vi "AnguloLimite.vi"(6 "XdoAttacker":dbl, 8 "atacando contra":bool, 9 "AnguloGol":dbl, 10 "IA State":T1={"our_robots"=[], "enemy_robots"=[], "balls"=[], "geometry"={"line_width"=0, "field_length"=0, "field_width"=0, "boundary_width"=0, "referee_width"=0, "goal_width"=0, "goal_depth"=0, "goal_wall_width"=0, "center_circle_radius"=0, "defense_radius"=0, "defense_stretch"=0, "free_kick_from_defense_dist"=0, "penalty_spot_from_field_line_dist"=0, "penalty_line_from_spot_dist"=0}, "IA Judge"={"stage"="", "command"="", "our_goalie_id"=0.0, "enemy_goalie_id"=0.0, "command enum"=enum."Halt", "Time"=enum."Azul"}, "Received Timestamp"=timestamp(0 s since 1904-01-01), "Events"={"Touch"=FALSE, "Ball out"=FALSE, "id touch"=0.0, "Ball out of \nVision"=FALSE, "Ball inside \nGoalie area"=FALSE, "Robot not responding"=FALSE, "Robots responding status"=[1.0, 1.0, 1.0, 1.0, 1.0, 1.0], "Enemy Ball \nPossession"=FALSE, "Pass State"=FALSE, "id end of pass"=0.0, "Kick"=FALSE, "Id ini Possession"=0.0, "Ball Possesion"=FALSE, "Id Possesion"=0.0}}, 11 "YdoAttacker":dbl) -> (1 "Angulo Limite":dbl)   [LabVIEW 2016]
uses:
  Core/AI Input.ctl
  Core/AI Robot.ctl
  Intel/Functions Enum.ctl
  Intel/AttackerStates.ctl
  Core/AI Ball.ctl
  Core/Field Size.ctl
  Core/AI Judge.ctl
  Intel/Command Enum.ctl
  Events/Events.ctl
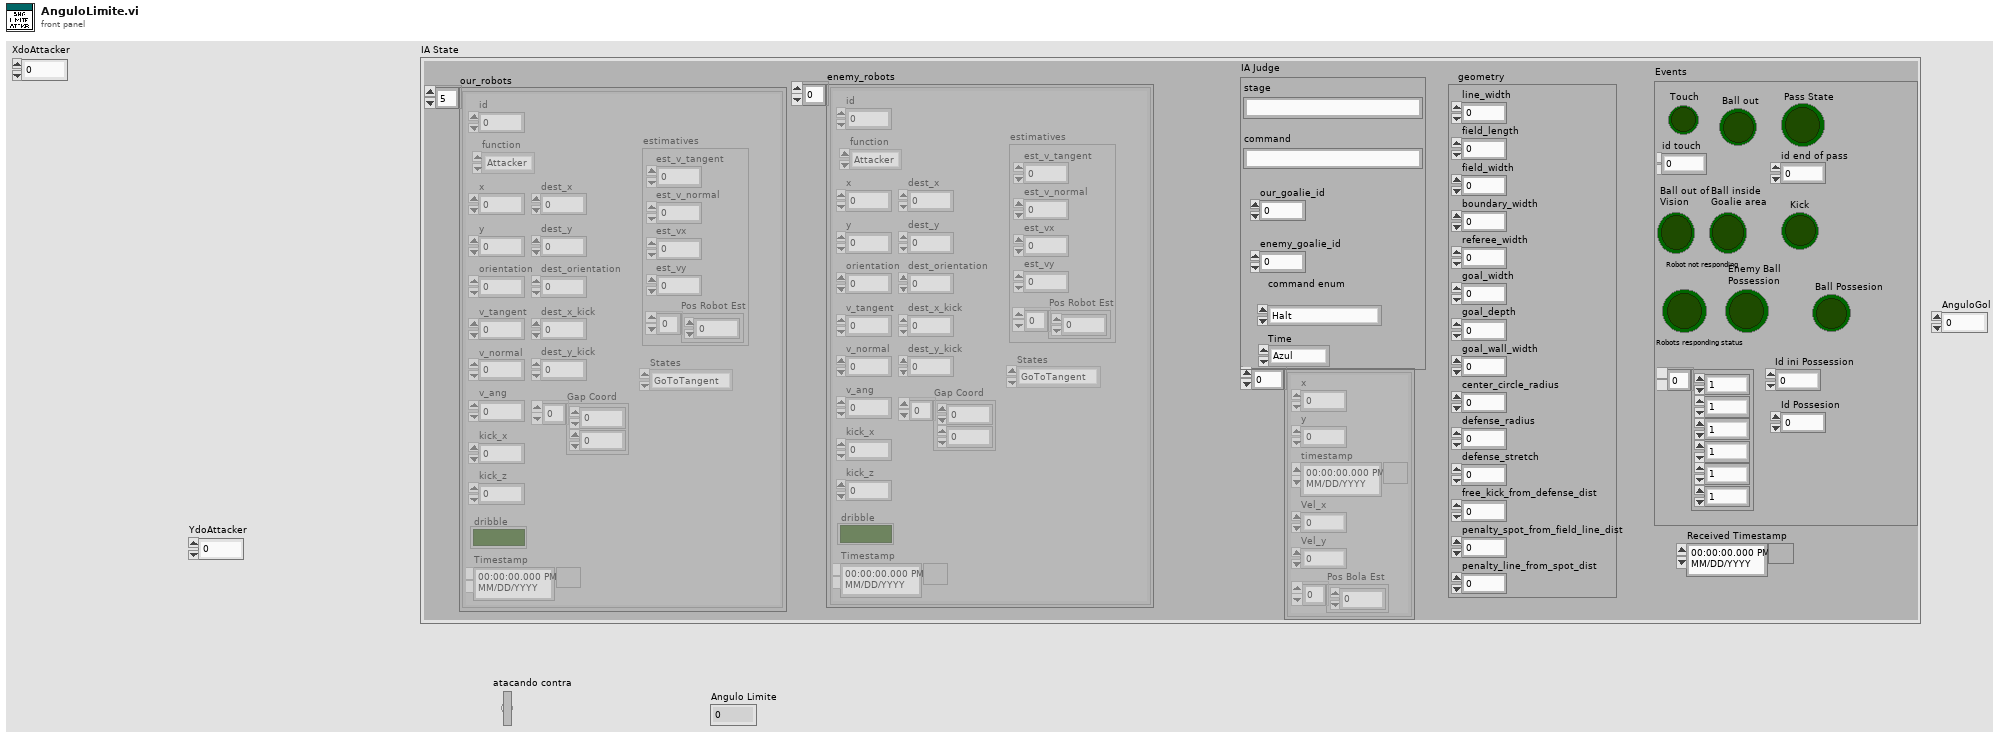
[diagram p1: front panel]
types:
  T1 = typedef "AI Input.ctl" = cluster{"our_robots":T2[], "enemy_robots":T2[], "balls":T5[], "geometry":T6, "IA Judge":T7, "Received Timestamp":timestamp, "Events":T9}
  T2 = typedef "AI Robot.ctl" = cluster{"id":u32, "function":T3, "x":dbl, "y":dbl, "orientation":dbl, "v_tangent":dbl, "v_normal":dbl, "v_ang":dbl, "kick_x":dbl, "kick_z":dbl, "dribble":bool, "Timestamp":timestamp, "dest_x":dbl, "dest_y":dbl, "dest_orientation":dbl, "estimatives":cluster{"est_v_tangent":dbl, "est_v_normal":dbl, "est_vx":dbl, "est_vy":dbl, "Pos Robot Est":dbl[]}, "dest_x_kick":dbl, "dest_y_kick":dbl, "Gap Coord":dbl[], "States":T4}
  T3 = typedef "Functions Enum.ctl" = enum16{"Attacker", "Goalie", "Defender", "Striker", "Goto 0", "Dummy", "Kicker", "ZigZag"}
  T4 = typedef "AttackerStates.ctl" = enum16{"Pass", "GoToTangent", "BallGetting", "GoToKick", ""}
  T5 = typedef "AI Ball.ctl" = cluster{"x":dbl, "y":dbl, "timestamp":timestamp, "Vel_x":dbl, "Vel_y":dbl, "Pos Bola Est":dbl[]}
  T6 = typedef "Field Size.ctl" = cluster{"line_width":u32, "field_length":u32, "field_width":u32, "boundary_width":u32, "referee_width":u32, "goal_width":u32, "goal_depth":u32, "goal_wall_width":u32, "center_circle_radius":u32, "defense_radius":u32, "defense_stretch":u32, "free_kick_from_defense_dist":u32, "penalty_spot_from_field_line_dist":u32, "penalty_line_from_spot_dist":u32}
  T7 = typedef "AI Judge.ctl" = cluster{"stage":string, "command":string, "our_goalie_id":dbl, "enemy_goalie_id":dbl, "command enum":T8, "Time":enum16{"Azul", "Amarelo"}}
  T8 = typedef "Command Enum.ctl" = enum16{"Halt", "Stop", "Force Start", "PKA Normal Start", "Prepare Kickoff Ally", "PKE Normal Start", "Prepare Kickoff Enemy", "Prepare Penalty Ally", "PPA Normal Start", "Prepare Penalty Enemy", "PPE Normal Start", "Direct Free Enemy", "Direct Free Ally", "Indirect Free Enemy", "Indirect Free Ally", "Timeout Enemy", "Timeout Ally", "Goal Enemy", "Goal Ally", "Ball Placement Enemy", "Ball Placement Ally", "Normal Half Time", "Extra Time Break", "Extra Half Time", "None", "Post Game"}
  T9 = typedef "Events.ctl" = cluster{"Touch":bool, "Ball out":bool, "id touch":dbl, "Ball out of \nVision":bool, "Ball inside \nGoalie area":bool, "Robot not responding":bool, "Robots responding status":dbl[], "Enemy Ball \nPossession":bool, "Pass State":bool, "id end of pass":dbl, "Kick":bool, "Id ini Possession":dbl, "Ball Possesion":bool, "Id Possesion":dbl}
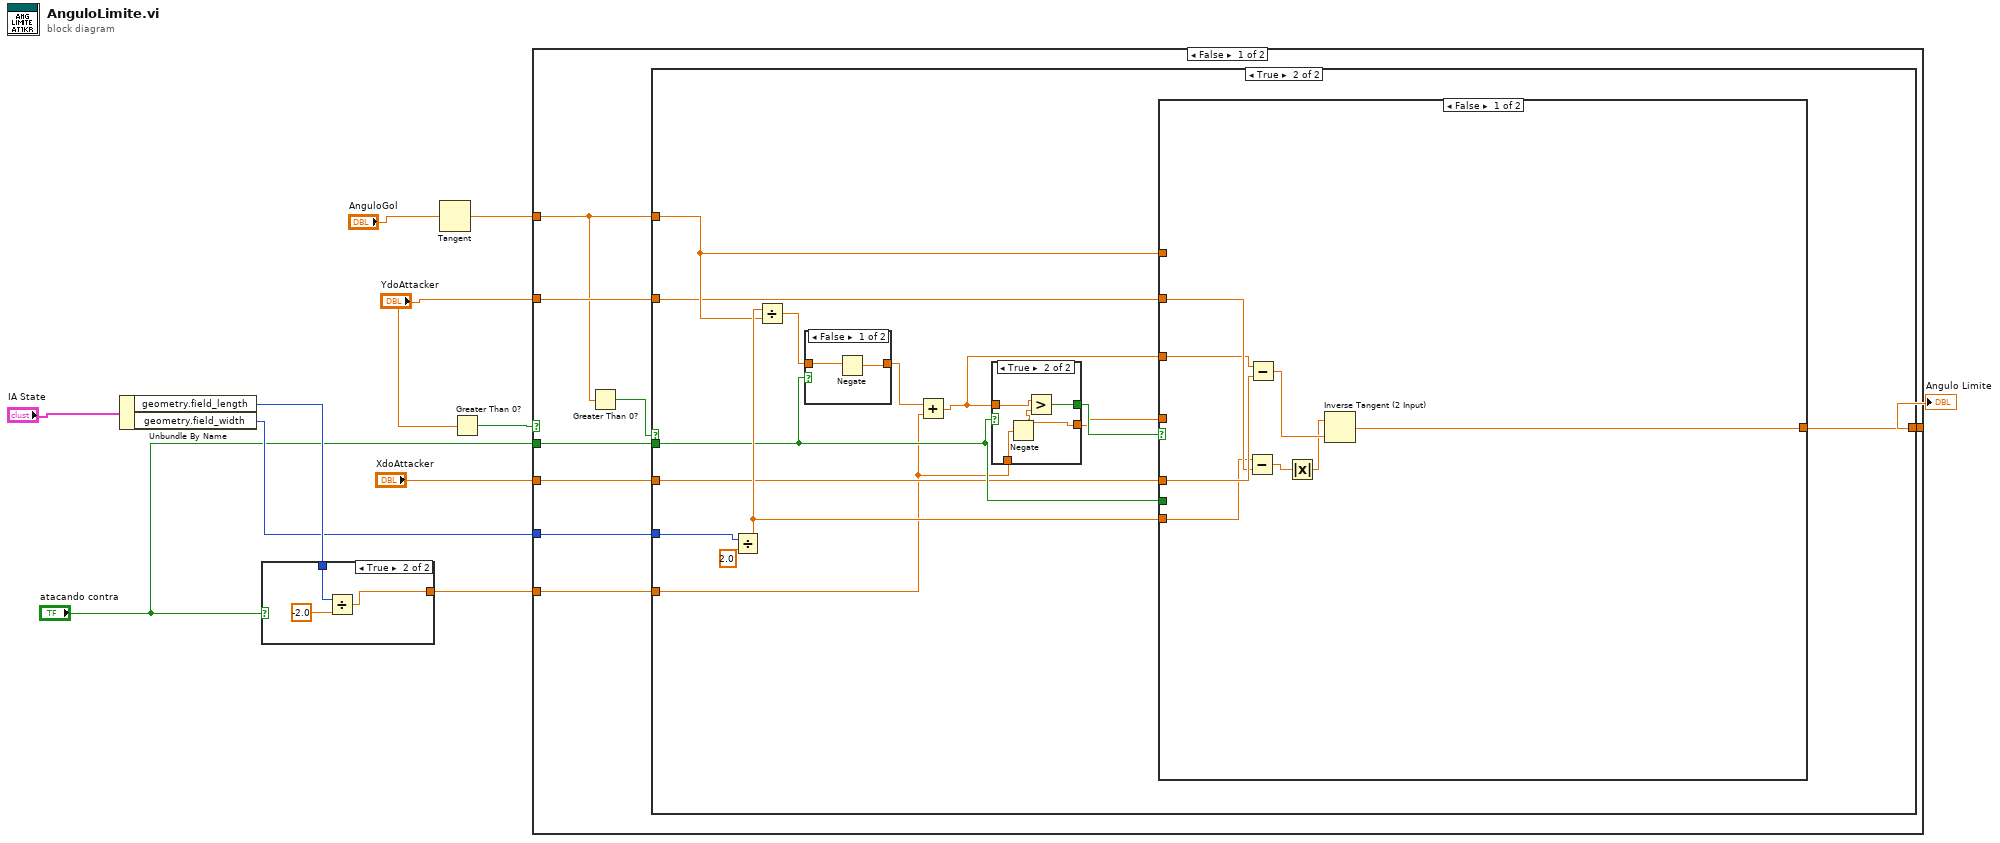
[diagram p0: block diagram]
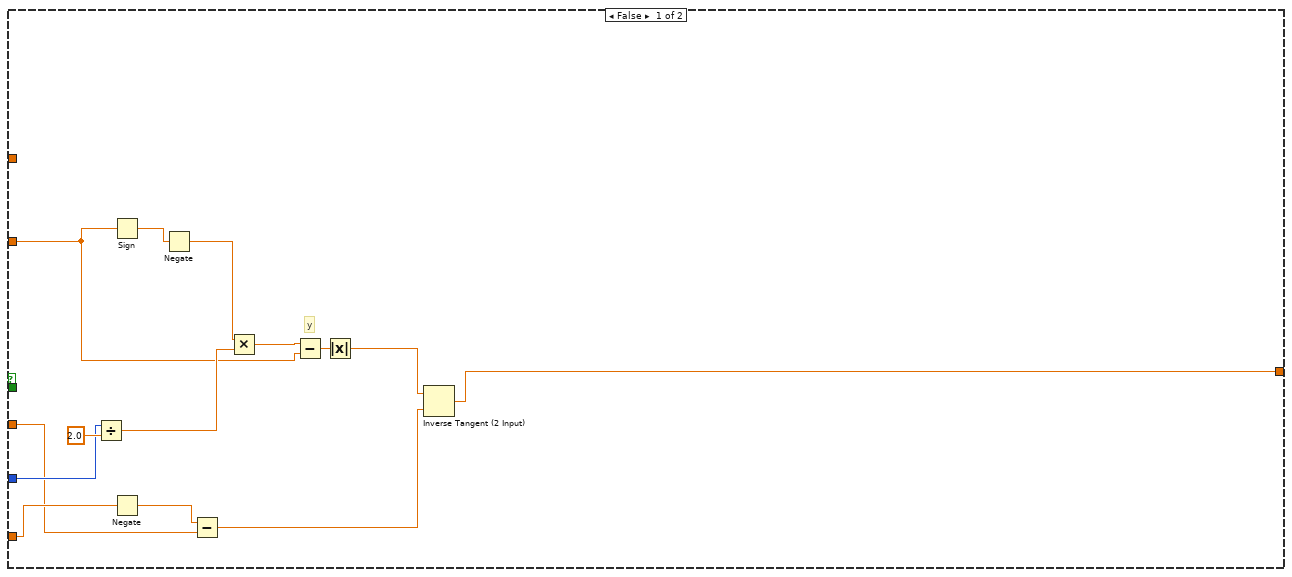
[diagram p2: hidden frame]
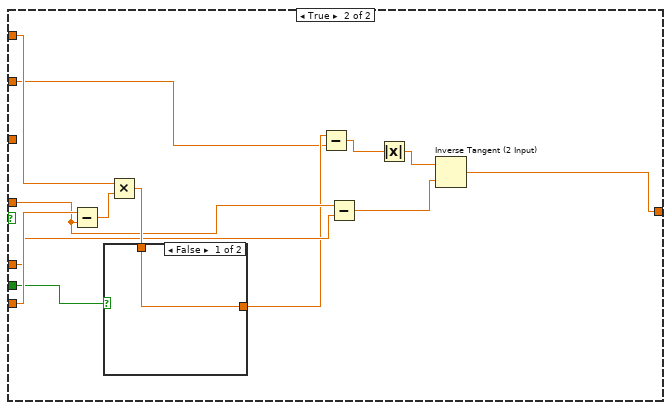
[diagram p3: hidden frame]
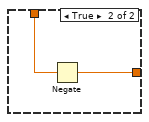
[diagram p4: hidden frame]
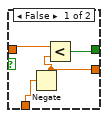
[diagram p5: hidden frame]
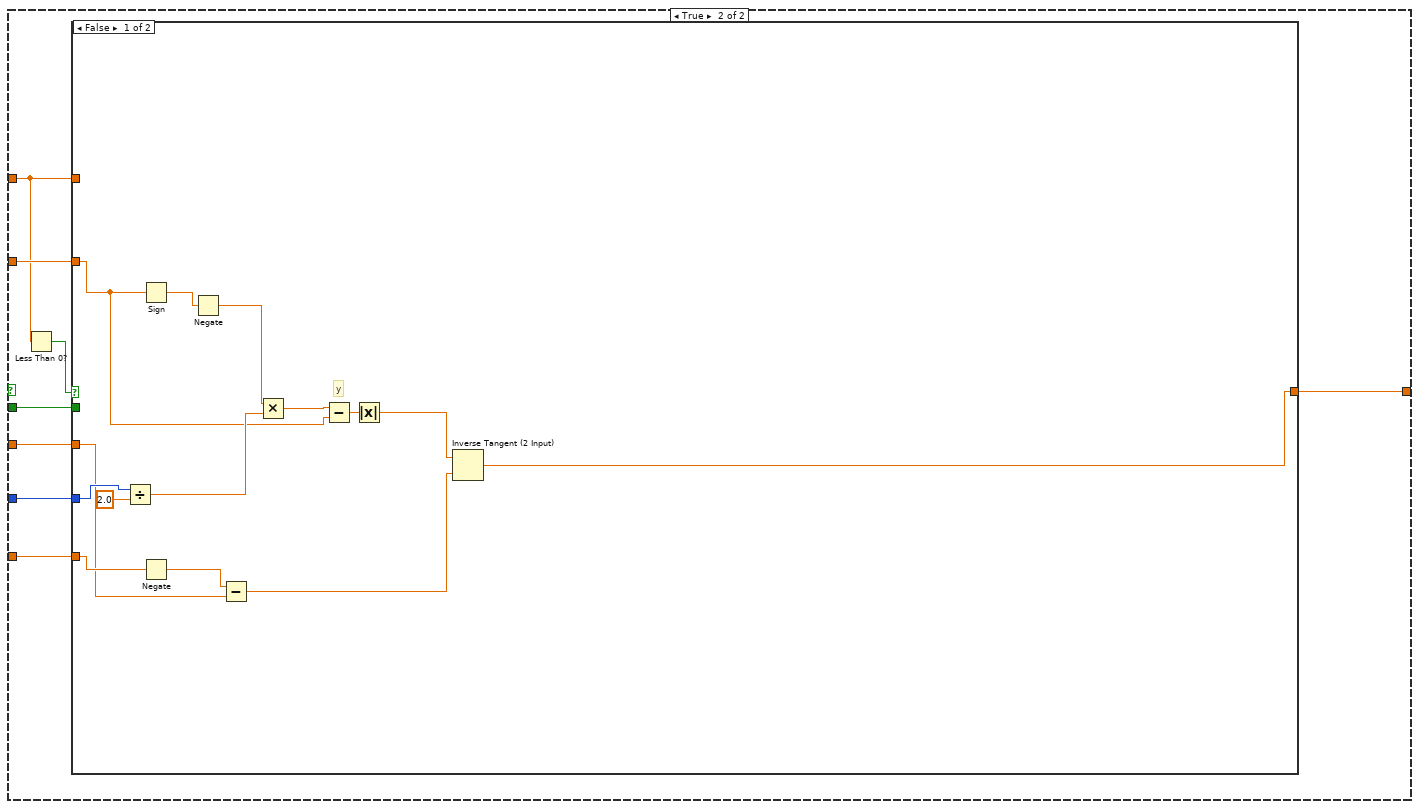
[diagram p7: hidden frame]
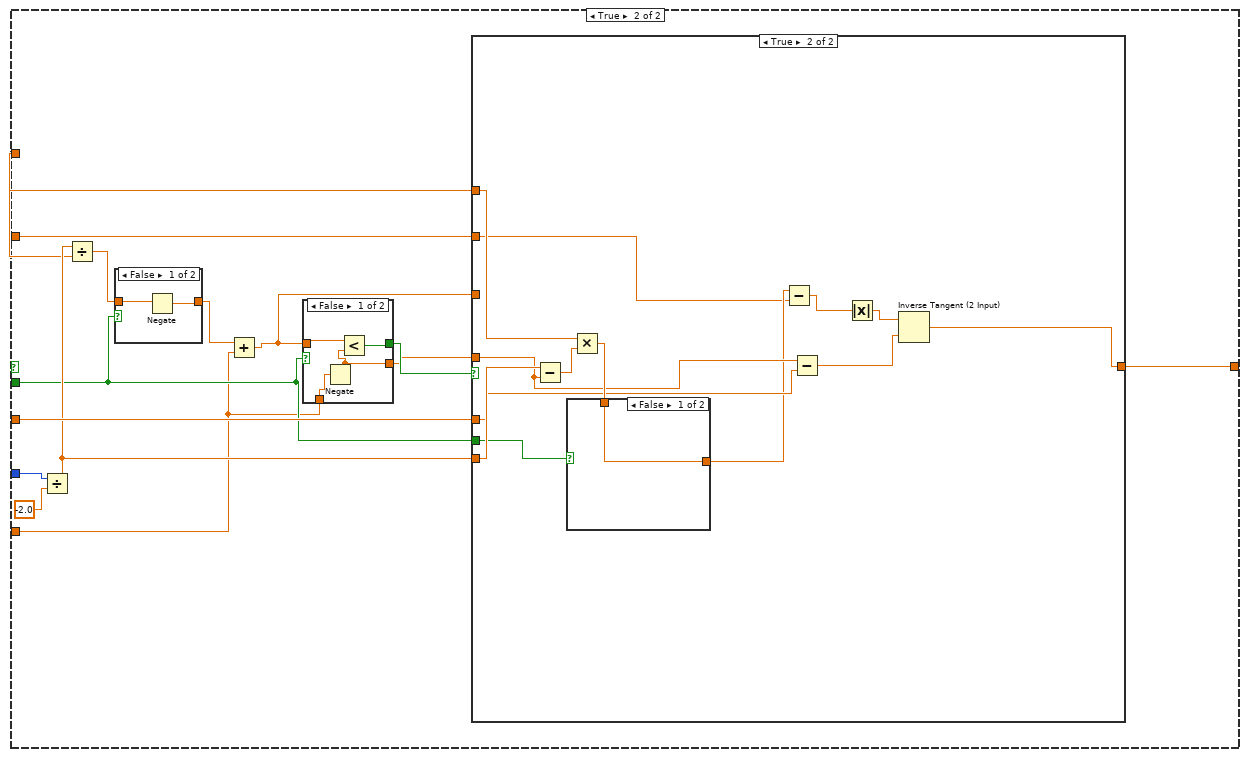
[diagram p8: hidden frame]
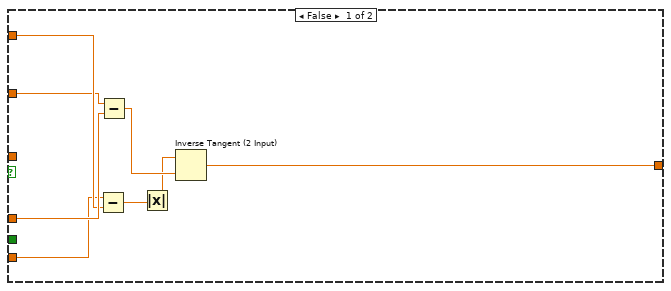
[diagram p9: hidden frame]
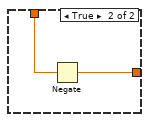
[diagram p10: hidden frame]
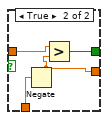
[diagram p11: hidden frame]
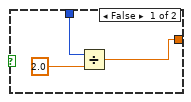
[diagram p13: hidden frame]
diagram:
  n1 = Unbundle By Name("IA State") -> ("geometry.field_length"=w10:u32, "geometry.field_width"=w8:u32)
  n2 = case shown="True" "atacando contra" {
    tunnel: w10 -> [w13 w17]
    tunnel: [w12 w15] -> w4
    frame False {
      n3 = Divide(x=w13, y=2.0) -> (x/y=w12:dbl)
    }
    frame True {
      n4 = Divide(x=w17, y=-2.0) -> (x/y=w15:dbl)
    }
  }
  n5 = Tangent(1:"AnguloGol") -> (0:w6:dbl)
  n6 = Greater Than 0?(x="YdoAttacker") -> (x > 0?=w9:bool)
  n7 = case shown="False" w9 {
    tunnel: w8 -> [w22 w96]
    tunnel: w6 -> [w20 w89]
    tunnel: "atacando contra" -> [w24 w92]
    tunnel: w4 -> [w21 w91]
    tunnel: "XdoAttacker" -> [w23 w95]
    tunnel: "YdoAttacker" -> [w25 w94]
    tunnel: [w18 w93] -> w1
    frame False {
      n8 = Greater Than 0?(x=w20) -> (x > 0?=w19:bool)
      n9 = case shown="True" w19 {
        tunnel: w20 -> [_ w46]
        tunnel: w25 -> [w30 w45]
        tunnel: w24 -> [_ w44]
        tunnel: w23 -> [w27 w43]
        tunnel: w22 -> [w29 w42]
        tunnel: w21 -> [w28 w41]
        tunnel: [w26 w40] -> w18
        frame False {
          # "y"
          n10 = Divide(x=w29, y=2.0) -> (x/y=w33:dbl)
          n11 = Sign(1:w30) -> (0:w31:dbl)
          n12 = Negate(x=w28) -> (-x=w36:dbl)
          n13 = Negate(x=w31) -> (-x=w34:dbl)
          n14 = Subtract(x=w36, y=w27) -> (x-y=w39:dbl)
          n15 = Multiply(x=w34, y=w33) -> (x*y=w35:dbl)
          n16 = Subtract(x=w35, y=w30) -> (x-y=w37:dbl)
          n17 = Absolute Value(x=w37) -> (abs(x)=w38:dbl)
          n18 = Inverse Tangent (2 Input)(1:w39, 2:w38) -> (0:w26:dbl)
        }
        frame True {
          n19 = Divide(x=w42, y=2.0) -> (x/y=w48:dbl)
          n20 = Divide(x=w48, y=w46) -> (x/y=w52:dbl)
          n21 = case shown="False" w44 {
            tunnel: w52 -> [w86 w88]
            tunnel: [w87 w88] -> w51
            frame False {
              n22 = Negate(x=w86) -> (-x=w87:dbl)
            }
            frame True {
            }
          }
          n23 = Add(x=w51, y=w41) -> (x+y=w49:dbl)
          n24 = case shown="True" w44 {
            tunnel: w49 -> [w80 w85]
            tunnel: w41 -> [w81 w84]
            tunnel: [w79 w83] -> w50
            tunnel: [w78 w82] -> w47
            frame False {
              n25 = Negate(x=w81) -> (-x=w78:dbl)
              n26 = Less?(x=w80, y=w78) -> (x < y?=w79:bool)
            }
            frame True {
              n27 = Negate(x=w84) -> (-x=w82:dbl)
              n28 = Greater?(x=w85, y=w82) -> (0:w83:bool)
            }
          }
          n29 = case shown="False" w50 {
            tunnel: w43 -> [w61 w68]
            tunnel: w45 -> [w60 w66]
            tunnel: w49 -> [w59 _]
            tunnel: w48 -> [w58 w74]
            tunnel: [w56 w65] -> w40
            tunnel: w46 -> [_ w72]
            tunnel: w47 -> [_ w69]
            tunnel: w44 -> [_ w71]
            frame False {
              n30 = Subtract(x=w58, y=w60) -> (x-y=w55:dbl)
              n31 = Subtract(x=w59, y=w61) -> (x-y=w57:dbl)
              n32 = Absolute Value(x=w55) -> (abs(x)=w54:dbl)
              n33 = Inverse Tangent (2 Input)(1:w57, 2:w54) -> (0:w56:dbl)
            }
            frame True {
              n34 = Subtract(x=w74, y=w69) -> (x-y=w73:dbl)
              n35 = Multiply(x=w72, y=w73) -> (x*y=w70:dbl)
              n36 = case shown="False" w71 {
                tunnel: w70 -> [w75 w77]
                tunnel: [w75 w76] -> w67
                frame False {
                }
                frame True {
                  n37 = Negate(x=w77) -> (-x=w76:dbl)
                }
              }
              n38 = Subtract(x=w67, y=w66) -> (x-y=w63:dbl)
              n39 = Subtract(x=w69, y=w68) -> (x-y=w64:dbl)
              n40 = Absolute Value(x=w63) -> (abs(x)=w62:dbl)
              n41 = Inverse Tangent (2 Input)(1:w64, 2:w62) -> (0:w65:dbl)
            }
          }
        }
      }
    }
    frame True {
      n42 = Less Than 0?(x=w89) -> (x < 0?=w90:bool)
      n43 = case shown="False" w90 {
        tunnel: w96 -> [w108 w124]
        tunnel: w95 -> [w101 w119]
        tunnel: w94 -> [w103 w118]
        tunnel: [w97 w115] -> w93
        tunnel: w89 -> [_ w114]
        tunnel: w92 -> [_ w112]
        tunnel: w91 -> [w105 w111]
        frame False {
          # "y"
          n44 = Divide(x=w108, y=2.0) -> (x/y=w107:dbl)
          n45 = Sign(1:w103) -> (0:w110:dbl)
          n46 = Negate(x=w105) -> (-x=w102:dbl)
          n47 = Negate(x=w110) -> (-x=w106:dbl)
          n48 = Subtract(x=w102, y=w101) -> (x-y=w98:dbl)
          n49 = Multiply(x=w106, y=w107) -> (x*y=w104:dbl)
          n50 = Subtract(x=w104, y=w103) -> (x-y=w100:dbl)
          n51 = Absolute Value(x=w100) -> (abs(x)=w99:dbl)
          n52 = Inverse Tangent (2 Input)(1:w98, 2:w99) -> (0:w97:dbl)
        }
        frame True {
          n53 = Divide(x=w124, y=-2.0) -> (x/y=w116:dbl)
          n54 = Divide(x=w116, y=w114) -> (x/y=w122:dbl)
          n55 = case shown="False" w112 {
            tunnel: w122 -> [w157 w159]
            tunnel: [w158 w159] -> w121
            frame False {
              n56 = Negate(x=w157) -> (-x=w158:dbl)
            }
            frame True {
            }
          }
          n57 = Add(x=w121, y=w111) -> (x+y=w117:dbl)
          n58 = case shown="False" w112 {
            tunnel: w117 -> [w151 w156]
            tunnel: w111 -> [w152 w155]
            tunnel: [w150 w154] -> w120
            tunnel: [w149 w153] -> w113
            frame False {
              n59 = Negate(x=w152) -> (-x=w149:dbl)
              n60 = Less?(x=w151, y=w149) -> (x < y?=w150:bool)
            }
            frame True {
              n61 = Negate(x=w155) -> (-x=w153:dbl)
              n62 = Greater?(x=w156, y=w153) -> (0:w154:bool)
            }
          }
          n63 = case shown="True" w120 {
            tunnel: w119 -> [w132 w139]
            tunnel: w118 -> [w131 w137]
            tunnel: w117 -> [w130 _]
            tunnel: w116 -> [w129 w145]
            tunnel: [w127 w136] -> w115
            tunnel: w114 -> [_ w143]
            tunnel: w113 -> [_ w140]
            tunnel: w112 -> [_ w142]
            frame False {
              n64 = Subtract(x=w129, y=w131) -> (x-y=w126:dbl)
              n65 = Subtract(x=w130, y=w132) -> (x-y=w128:dbl)
              n66 = Absolute Value(x=w126) -> (abs(x)=w125:dbl)
              n67 = Inverse Tangent (2 Input)(1:w128, 2:w125) -> (0:w127:dbl)
            }
            frame True {
              n68 = Subtract(x=w145, y=w140) -> (x-y=w144:dbl)
              n69 = Multiply(x=w143, y=w144) -> (x*y=w141:dbl)
              n70 = case shown="False" w142 {
                tunnel: w141 -> [w146 w148]
                tunnel: [w146 w147] -> w138
                frame False {
                }
                frame True {
                  n71 = Negate(x=w148) -> (-x=w147:dbl)
                }
              }
              n72 = Subtract(x=w138, y=w137) -> (x-y=w133:dbl)
              n73 = Subtract(x=w140, y=w139) -> (x-y=w135:dbl)
              n74 = Absolute Value(x=w133) -> (abs(x)=w134:dbl)
              n75 = Inverse Tangent (2 Input)(1:w135, 2:w134) -> (0:w136:dbl)
            }
          }
        }
      }
    }
  }
  "Angulo Limite" <- w1
